vi "initialise tasks.vi"(8 "error in (no error)":errorcluster, 11 "Waveform in":refnum<class "Waveform.lvclass">) -> (0 "error out":errorcluster, 3 "Waveform out":refnum<class "Waveform.lvclass">)   [LabVIEW 2012, in "Waveform.lvclass"]
uses:
  Waveform.lvclass
  Waveform.lvclass/Waveform.ctl
  <vilib>/DAQmx/write.llb/DAQmx Write (Digital 1D Bool 1Chan 1Samp).vi
  <vilib>/DAQmx/create/channels.llb/DAQmx Create Channel (AO-Voltage-Basic).vi
  <vilib>/DAQmx/create/channels.llb/DAQmx Create Channel (CO-Pulse Generation-Frequency).vi
  <vilib>/DAQmx/create/channels.llb/DAQmx Create Channel (DO-Digital Output).vi
  <vilib>/DAQmx/miscellaneous.llb/DAQmx Fill In Error Info.vi
  <resource>/objmgr/daqmx.rc
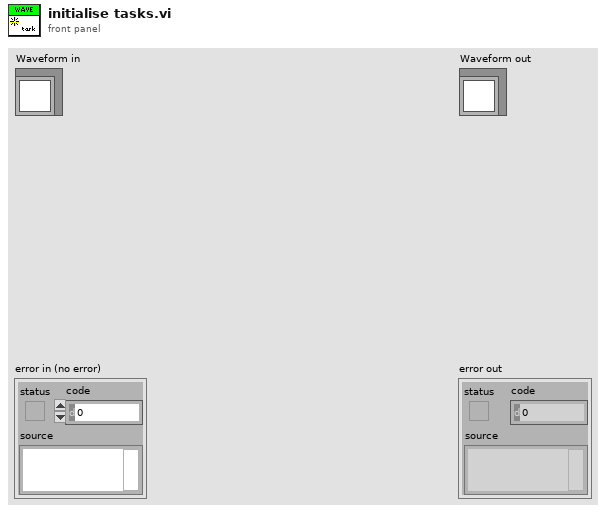
[diagram p1: front panel]
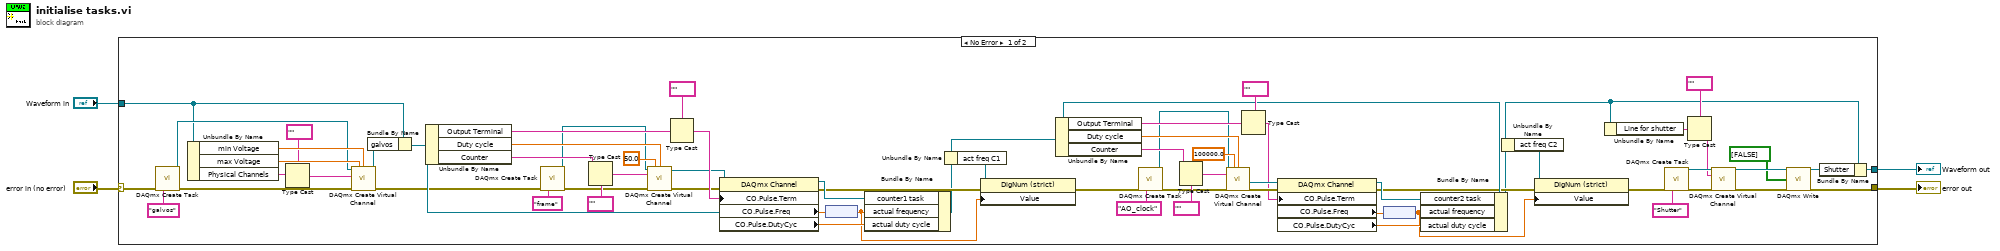
[diagram p0: block diagram]
diagram:
  n1 = case shown="No Error" "error in (no error)" {
    selector: "error in (no error)" -> [w30 w73]
    tunnel: [w12 w73] -> w3
    tunnel: [w8 w72] -> w1
    tunnel: "Waveform in" -> [w31 w72]
    frame No Error {
      n2 = call <vilib>:"DAQmx Create Task.vi"("new task name"="galvos", "error in"=w30) -> ("task out"=w38:refnum<k21>, "error out"=w40:errorcluster)  [unwired: 12 in]
      n3 = Unbundle By Name(w31) -> ("min Voltage"=w70:dbl, "max Voltage"=w71:dbl, "Physical Channels"=w59:string)
      n4 = Type Cast(type=tag "" ("physical channels"), x=w59) -> (*(type *) &x=w41:tag)
      n5 = call-poly <vilib>:"DAQmx Create Virtual Channel.vi"("task in"=w38, "maximum value"=w71, "minimum value"=w70, "physical channels"=w41, "error in"=w40) -> ("task out"=w29:refnum<k21>, "error out"=w5:errorcluster)  [unwired: 9 in]
      n6 = Bundle By Name(cluster=w31, "galvos"=w29) -> (w6:refnum<class "Waveform.lvclass">)
      n7 = Unbundle By Name(w6) -> ("Output Terminal"=w53:string, "Duty cycle"=w69:dbl, "Counter"=w57:string)
      n8 = call <vilib>:"DAQmx Create Task.vi"("new task name"="frame", "error in"=w5) -> ("task out"=w36:refnum<k21>, "error out"=w37:errorcluster)  [unwired: 12 in]
      n9 = Type Cast(type=tag "" ("counter"), x=w57) -> (*(type *) &x=w56:tag)
      n10 = call-poly <vilib>:"DAQmx Create Virtual Channel.vi"("task in"=w36, "frequency"=50.0, "duty cycle"=w69, "counter"=w56, "error in"=w37) -> ("task out"=w45:refnum<k21>, "error out"=w44:errorcluster)  [unwired: 9 in]
      n11 = Type Cast(type=tag "" ("CO.Pulse.Term"), x=w53) -> (*(type *) &x=w52:tag)
      n12 = property class="DAQmx Channel"(reference=w45, error in=w44, "CO.Pulse.Term"=w52) -> (reference out=w68:refnum<k21>, error out=w28:errorcluster, "CO.Pulse.Freq"=w67:dbl, "CO.Pulse.DutyCyc"=w66:dbl)
      n13 = node(w67) -> (w24:dbl[unit])
      n14 = Bundle By Name(cluster=w6, "counter1 task"=w68, "actual frequency"=w24, "actual duty cycle"=w66) -> (w26:refnum<class "Waveform.lvclass">)
      n15 = Unbundle By Name(w26) -> ("act freq C1"=w25:refnum<vi>)
      n16 = property class="DigNum (strict)"(reference=w25, error in=w28, "Value"=w24) -> (error out=w27:errorcluster)  [unwired: 1 out]
      n17 = Unbundle By Name(w26) -> ("Output Terminal"=w51:string, "Duty cycle"=w60:dbl, "Counter"=w48:string)
      n18 = call <vilib>:"DAQmx Create Task.vi"("new task name"="AO_clock", "error in"=w27) -> ("task out"=w33:refnum<k21>, "error out"=w34:errorcluster)  [unwired: 12 in]
      n19 = Type Cast(type=tag "" ("counter"), x=w48) -> (*(type *) &x=w46:tag)
      n20 = call-poly <vilib>:"DAQmx Create Virtual Channel.vi"("task in"=w33, "frequency"=100000.0, "duty cycle"=w60, "counter"=w46, "error in"=w34) -> ("task out"=w62:refnum<k21>, "error out"=w61:errorcluster)  [unwired: 9 in]
      n21 = Type Cast(type=tag "" ("CO.Pulse.Term"), x=w51) -> (*(type *) &x=w50:tag)
      n22 = property class="DAQmx Channel"(reference=w62, error in=w61, "CO.Pulse.Term"=w50) -> (reference out=w63:refnum<k21>, error out=w23:errorcluster, "CO.Pulse.Freq"=w64:dbl, "CO.Pulse.DutyCyc"=w65:dbl)
      n23 = node(w64) -> (w21:dbl[unit])
      n24 = Bundle By Name(cluster=w26, "counter2 task"=w63, "actual frequency"=w21, "actual duty cycle"=w65) -> (w9:refnum<class "Waveform.lvclass">)
      n25 = Unbundle By Name(w9) -> ("act freq C2"=w22:refnum<vi>)
      n26 = property class="DigNum (strict)"(reference=w22, error in=w23, "Value"=w21) -> (error out=w20:errorcluster)  [unwired: 1 out]
      n27 = Unbundle By Name(w9) -> ("Line for shutter"=w16:string)
      n28 = call <vilib>:"DAQmx Create Task.vi"("new task name"="Shutter", "error in"=w20) -> ("task out"=w17:refnum<k21>, "error out"=w18:errorcluster)  [unwired: 12 in]
      n29 = Type Cast(type=tag "" ("lines"), x=w16) -> (*(type *) &x=w14:tag)
      n30 = call-poly <vilib>:"DAQmx Create Virtual Channel.vi"("task in"=w17, "lines"=w14, "error in"=w18) -> ("task out"=w11:refnum<k21>, "error out"=w13:errorcluster)  [unwired: 11 in]
      n31 = call-poly <vilib>:"DAQmx Write.vi"("task/channels in"=w11, "data"=bool[] [FALSE], "error in"=w13) -> ("task out"=w7:refnum<k21>, "error out"=w12:errorcluster)  [unwired: 10 in, 1 out]
      n32 = Bundle By Name(cluster=w9, "Shutter"=w7) -> (w8:refnum<class "Waveform.lvclass">)
    }
    frame Error {
    }
  }
  "error out" <- w3
  "Waveform out" <- w1
